vi "Get Attributes.vi"(8 "error in (no error)":errorcluster, 11 "For Loop Dialog in":refnum<class "Subroutine Dialog.lvclass">) -> (0 "error out":errorcluster, 3 "For Loop Dialog out":refnum<class "Subroutine Dialog.lvclass">)   [LabVIEW 2020, in "Subroutine Dialog.lvclass"]
uses:
  <vilib>/gpm_packages/@cs/Test-executive-builder/Source/Test Executive Builder Dialogs/Edit Subroutine Dialog/Subroutine Dialog.lvclass
  C:/Program Files/National Instruments/LabVIEW 2020/vi.lib/gpm_packages/@cs/Test-executive-builder/Source/Test Executive Builder Dialogs/ITest Executive Builder Dialog/ITest Executive Builder Dialog.lvclass
  <vilib>/gpm_packages/@cs/Test-executive-builder/Source/Test Executive Builder Dialogs/ITest Executive Builder Dialog/ITest Executive Builder Dialog.lvclass/ITest Executive Builder Dialog.ctl
  <vilib>/gpm_packages/@cs/Test-executive-builder/Source/Test Executive Builder Dialogs/Edit Subroutine Dialog/Subroutine Dialog.lvclass/Subroutine Dialog.ctl
  191dc990-9661-4c30-b313-8302c425e24e.vi
  bd3c3d9a-c639-4d3a-a825-43e3a07e4ab5.vi
  a0e6a74e-5798-41ce-a401-da88ee2081e3.vi
  <vilib>/Utility/error.llb/Clear Errors.vi
  <vilib>/gpm_packages/@cs/test-executive/Source/Test Executive/ITestExecutive/ITest Executive.lvclass
  <vilib>/gpm_packages/@cs/Test-executive-builder/Source/Data Type Handler/Test Executive Builder Data Type Handler.lvclass
  <vilib>/gpm_packages/@cs/Test-executive-builder/Source/Test Executive Builder Dialogs/ITest Executive Builder Dialog/ITest Executive Builder Dialog.lvclass
  <vilib>/gpm_packages/@cs/test-executive/Source/Test Executive/TestExecutive Ref/TestExecutive Ref.lvclass
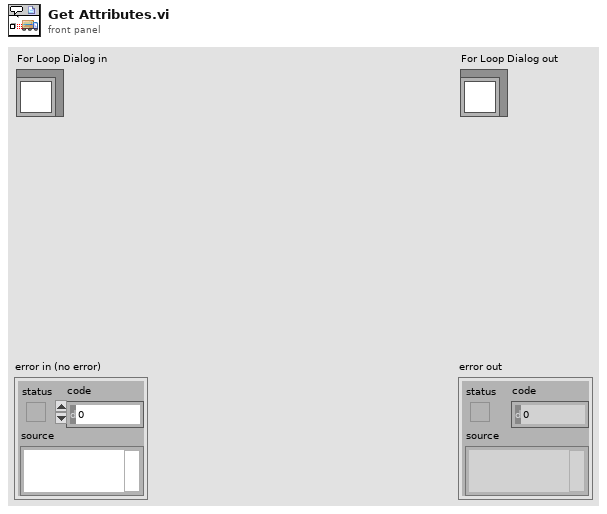
[diagram p1: front panel]
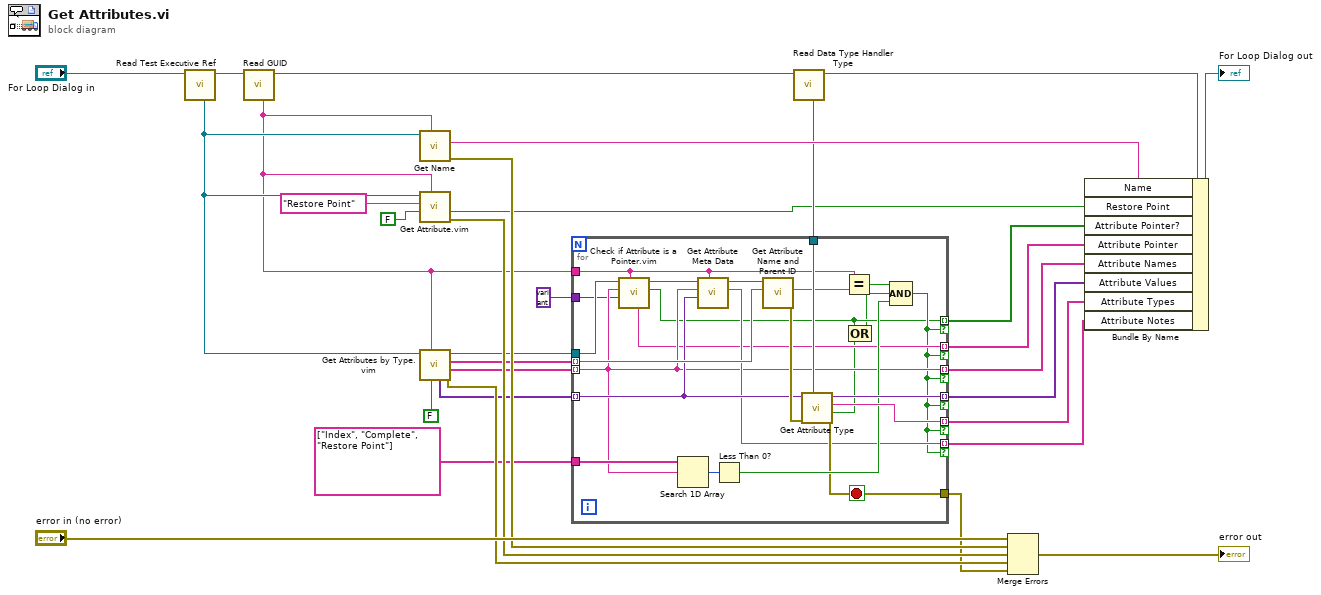
[diagram p0: block diagram]
diagram:
  n1 = call <vilib>:"Read Test Executive Ref.vi"("ITest Executive Builder Dialog in"="For Loop Dialog in") -> ("ITest Executive Builder Dialog out"=w30:refnum<class "Subroutine Dialog.lvclass">, "Test Executive Ref"=w21:refnum<data-value>)  [unwired: 9 in]
  n2 = call <vilib>:"Read GUID.vi"("ITest Executive Builder Dialog in"=w30) -> ("ITest Executive Builder Dialog out"=w13:refnum<class "Subroutine Dialog.lvclass">, "GUID"=w14:string)  [unwired: 9 in]
  n3 = call <vilib>:"Get Name.vi"("Unique ID"=w14, "Test Executive Ref"=w21) -> ("error out"=w22:errorcluster, "Name"=w29:string)  [unwired: 5 in, 3 out]
  n4 = call "Get Attribute.vim"("ID"=w14, "Type"=FALSE, "Attribute Name"="Restore Point", "Test Executive Ref"=w21) -> ("error out"=w23:errorcluster, "Attribute"=w9:bool)  [unwired: 3 in, 3 out]
  n5 = call "Get Attributes by Type.vim"("Recurse Up List (Default=True)"=FALSE, "ID"=w14, "Test Executive Ref"=w21) -> ("error out"=w20:errorcluster, "Names"=w17:string[], "IDs"=w16:string[], "Test Executive Ref out"=w15:refnum<data-value>, "Attributes"=w18:variant[])  [unwired: 4 in]
  n6 = call <vilib>:"Read Data Type Handler Type.vi"("ITest Executive Builder Dialog in"=w13) -> ("ITest Executive Builder Dialog out"=w12:refnum<class "Subroutine Dialog.lvclass">, "Data Type Handler"=w11:refnum<class "Test Executive Builder Data Type Handler.lvclass">)  [unwired: 9 in]
  n7 = for {
    tunnel: w18 -> [w43] mode=indexing
    tunnel: w17 -> [w38] mode=indexing
    tunnel: w16 -> [w55] mode=indexing
    tunnel: w15 -> [w41]
    tunnel: w14 -> [w39]
    tunnel: w11 -> [w54]
    tunnel: [w45] -> w10
    tunnel: [w38] -> w7 mode=indexing if=w36
    tunnel: [w52] -> w5 mode=indexing if=w36
    tunnel: [w49] -> w6 mode=indexing if=w36
    tunnel: string[] ["Index", "Complete", "Restore Point"] -> [w48]
    tunnel: [w42] -> w4 mode=indexing if=w36
    tunnel: [w37] -> w3 mode=indexing if=w36
    tunnel: [w34] -> w2 mode=indexing if=w36
    tunnel: variant -> [w35]
    stop <- w45 stop-if-true
    n8 = call "Check if Attribute is a Pointer.vim"("ID"=w39, "Type"=w35, "Attribute Name"=w38, "Test Executive Ref"=w41) -> ("Pointer?"=w34:bool, "Test Executive Ref out"=w40:refnum<data-value>, "Pointer ID"=w37:string)  [unwired: 3 in, 2 out]
    n9 = Search 1D Array(1D array=w48, element=w38) -> (index of element=w47:i32)  [unwired: 1 in]
    n10 = call <vilib>:"Get Attribute Meta Data.vi"("Unique ID"=w39, "Attribute Type"=w43, "Attribute Name"=w38, "Test Executive Ref"=w40) -> ("Meta Data"=w42:string, "Test Executive Ref out"=w44:refnum<data-value>)  [unwired: 4 in, 2 out]
    n11 = Less Than 0?(x=w47) -> (x < 0?=w46:bool)
    n12 = call <vilib>:"Get Attribute Name and Parent ID.vi"("Tag"=w55, "Test Executive Ref"=w44) -> ("error out"=w53:errorcluster, "Parent ID"=w51:string)  [unwired: 6 in, 2 out]
    n13 = call-dynamic "Get Attribute Type.vi"("Test Executive Builder Data Type Handler in"=w54, "error in (no error)"=w53, "Potential Attribute in"=w43) -> ("error out"=w45:errorcluster, "Valid Type?"=w33:bool, "Attribute Type"=w52:string, "Potential Attribute out"=w49:variant)  [unwired: 5 in]
    n14 = Equal?(x=w39, y=w51) -> (x = y?=w50:bool)
    n15 = Compound Arithmetic op=OR(w34, w33) -> (w32:bool)
    n16 = Compound Arithmetic op=AND(w50, w32, w46) -> (w36:bool)
  }
  n17 = Merge Errors("error in (no error)", w22, w23, w20, w10) -> (→"error out":errorcluster)
  n18 = Bundle By Name(cluster=w12, "Name"=w29, "Restore Point"=w9, "Attribute Pointer?"=w2, "Attribute Pointer"=w3, "Attribute Names"=w7, "Attribute Values"=w6, "Attribute Types"=w5, "Attribute Notes"=w4) -> (→"For Loop Dialog out":refnum<class "Subroutine Dialog.lvclass">)
